vi "MatrixHelper_MultCoerceBSize.vi"(9 "B":T1, 11 "A":T1) -> (0 "Coerced":bool, 3 "Updated B":T1)   [LabVIEW 2019, in "Trajectory_Library.lvlib"]
doc: "Ensure that the B matrix is the correct size before performing the matrix multiplication A x B.\n\nInputs:\n -- A -- A matrix\n -- B -- B matrix\n \nOutputs:\n - Updated B -- B matrix, resized as necessary to multiply with A.\n - Coerced -- If TRUE, the size of B was changed."
uses:
  Trajectory_Library.lvlib
  <vilib>/Analysis/Matrix/Datatypes/RealMatrix.ctl
  <vilib>/Analysis/Matrix/NI_Matrix.lvlib
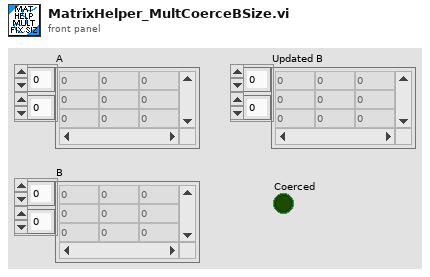
[diagram p1: front panel]
types:
  T1 = typedef "NI_Matrix.lvlib/RealMatrix.ctl" = dbl[][]
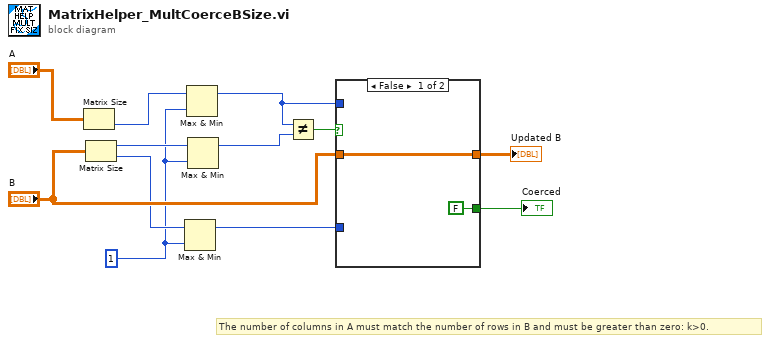
[diagram p0: block diagram]
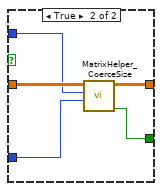
[diagram p2: hidden frame]
diagram:
  w2 = 1
  # "The number of columns in A must match the number of rows in B and must be greater than zero: k>0."
  n1 = Matrix Size(0:"A") -> (2:w8:i32)  [unwired: 1 out]
  n2 = Matrix Size(0:"B") -> (1:w5:i32, 2:w6:i32)
  n3 = Max & Min(x=w6, y=w2) -> (max(x,y)=w3:i32)  [unwired: 1 out]
  n4 = Max & Min(x=w8, y=w2) -> (max(x,y)=w7:i32)  [unwired: 1 out]
  n5 = Max & Min(x=w5, y=w2) -> (max(x,y)=w4:i32)  [unwired: 1 out]
  n6 = Not Equal?(x=w7, y=w4) -> (x != y?=w10:bool)
  n7 = case shown="False" w10 {
    tunnel: "B" -> [w14 w19]
    tunnel: w3 -> [_ w17]
    tunnel: w7 -> [_ w18]
    tunnel: [w14 w16] -> w12
    tunnel: [FALSE ("Coerced") w15] -> w1
    frame False {
    }
    frame True {
      n8 = call "MatrixHelper_CoerceSize.vi"("Columns"=w17, "Rows"=w18, "input matrix"=w19) -> ("Coerced"=w15:bool, "output matrix"=w16:T1)  [unwired: 7 in]
    }
  }
  "Updated B" <- w12
  "Coerced" <- w1
